vi "zlgcan_demo_CANFDNET_TCP .vi"() -> ()   [LabVIEW 2018]
doc: "适用的设备：CANET-E-U、CANET-2E-U、CANET-4E-U、CANET-8E-U、\nCANET-200T、CANET-100T"
uses:
  data_type/ZCAN_InitCAN_setting_CANET.ctl
  data_type/ZCAN_TransmitFD_Data.ctl
  data_type/ZCAN_Transmit_Data.ctl
panel:
  in  "ZCAN_Transmit_Data":T1
  in  "ZCAN_TransmitFD_Data":T2
  in  "CANFD数据帧数组":T3(array[cluster])
  in  "CAN数据帧数组":T4(array[cluster])
  out "已接收帧数":u32
  out "CAN报文显示":string[][](table)
  out "CANFD报文显示":string[][](table)
  out "error out 2":errorcluster caption="错误输出"
  out "source":string
  in  "ZCAN_InitCAN_setting_CANET":T5
  in  "开启CAN":bool
  in  "stop":bool
  in  "?":T6(tab)
  in  "CAN卡型号":u32(ring)=48 items=["CANFDNET-800U -TCP"=57, "CANFDNET-100U -TCP"=55, "CANFDNET-400U -TCP"=52, "CANFDNET-200U-TCP"=48]
  in  "索引":u32(ring) items=["0", "1", "2", "3", "4", "5", "6", "7", "8"]
  in  "CAN 通道":u32(ring) items=["0", "1", "2", "3"]
  in  "TCP模式":u32(ring) items=["客户端（client）", "服务器（server）"]
  in  "IP":string="192.168.0.178"
  in  "工作端口":u32=4001
  in  "本地端口":u32=8000
  out "设备句柄":u32
  out "通道句柄":u32
  out "error out":errorcluster caption="状态"
  out "数据长度":u8=8 max=8
  in  "CANFD加速？":u32(ring) items=["不加速", "加速"]
  in  "数据输入":string="11 22 33 44 55 66 77 88"
  in  "协议":u32(ring) items=["CAN", "CANFD"]
  in  "发送方式":u32(ring) items=["正常发送", "单次发送", "自发自收", "单次自发自收"]
  in  "帧格式":u32(ring) items=["数据帧", "远程帧"]
  in  "帧类型":u32(ring) items=["标准帧", "扩展帧"]
  in  "ID":u32=18 format="0x%08x"
  in  "发送":bool
  # "适用的设备：CANFDNET-100U -TCP、CANFDNET200U_TCP、CANFDNET-400U -TCP、CANFDNET-800U -TCP"
  # "停止程序前，\n请先关闭CAN卡"
  # "当CANET的工作模式为：\n\n1. 客户端（TCP Client）\n\n   LabVIEW 设备型号选择【 CANFDNET-TCP】\n\n   TCP模式选择【服务器 TCP Sever】\n\n   填写电脑本机IP+本地端口。\n\n2. 服务器（TCP Sever）\n\n   LabVIEW 设备型号选择【 CANFDNET-TCP】\n\n   TCP模式选择【客户端 TCP Client】\n\n   填写CANFDNET的 IP +工作端口\n\n3. UDP\n\n   LabVIEW 设备型号选择【 CANFDNET-UDP】\n\n   填写CANFDNET的IP+工作端口+本地端口"
  # "1. 调试运行DEMO前，将bin文件夹下面的kerneldlls文件夹先拷贝至LabView安装目录，\n如 D:\\Program Files (x86)\\National Instruments\\LabVIEW 2018。"
  # "2. 确保电脑有VC++ 2005/2008/2010/2013运行库（对应32，64位），可到微软官网下载。"
  # "3，如果打开设备失败，可能原因：\n（1）没有进行第二步操作；\n（2）已经打开过一次，没有正常关闭的情况下，继续点击“打开设备”，是无法打开的。\n     需要USB重新拔插，LABVIEW重启（全部关闭），然后再“打开设备”。\n (3) 项目路径不能有中文繁体。"
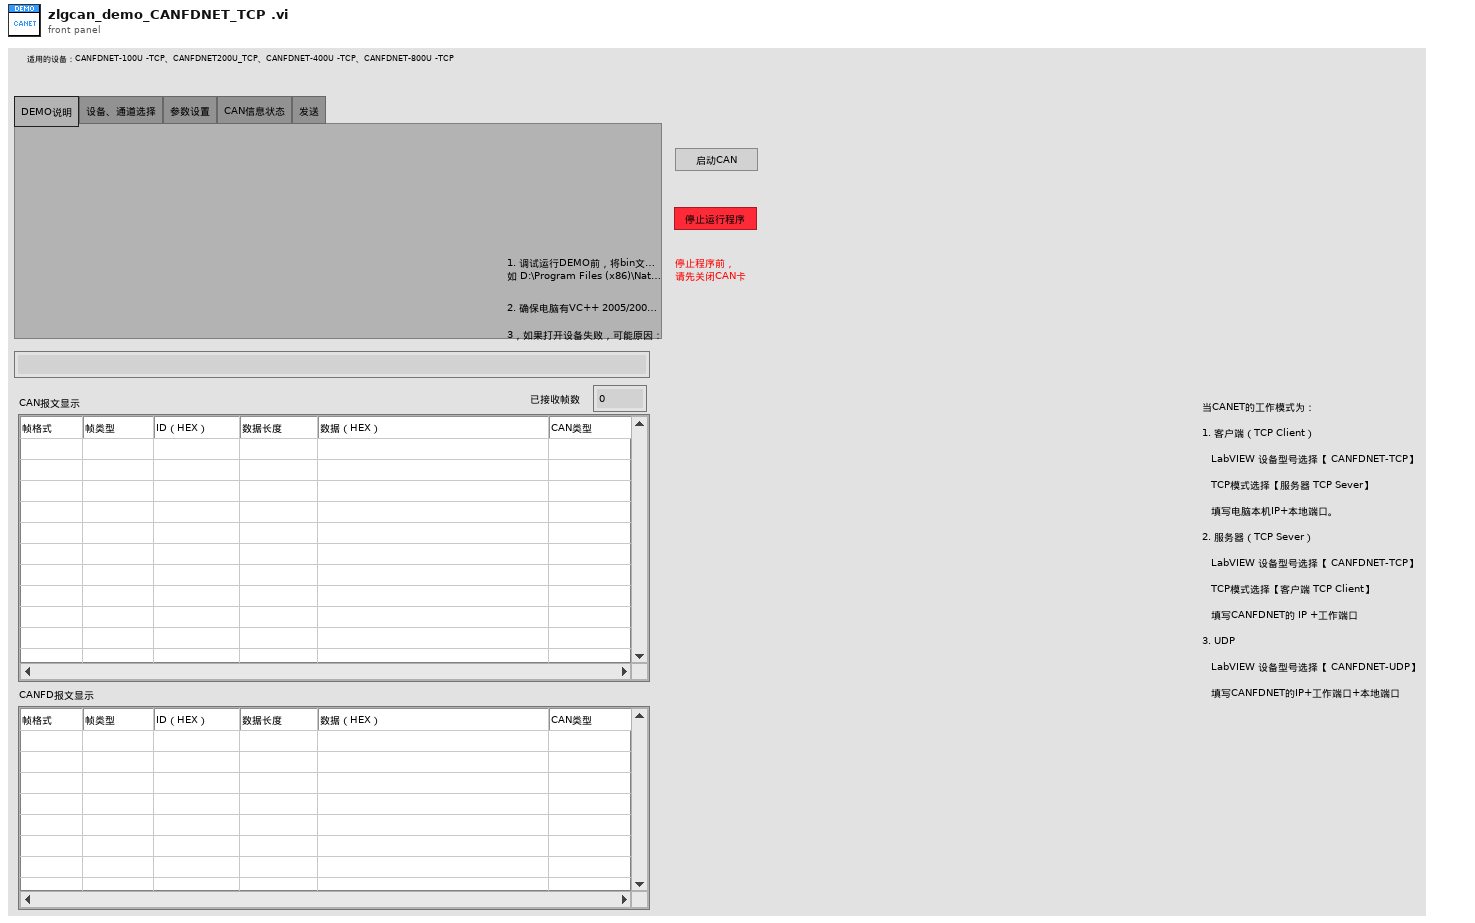
[diagram p1: front panel]
types:
  T1 = typedef "ZCAN_Transmit_Data.ctl" = cluster{"帧类型":u32, "帧格式":u32, "ID":u32, "数据长度":u8, "DATA":cluster{"CAN数据[0]":u8, "CAN数据[1]":u8, "CAN数据[2]":u8, "CAN数据[3]":u8, "CAN数据[4]":u8, "CAN数据[5]":u8, "CAN数据[6]":u8, "CAN数据[7]":u8}, "发送方式":u32}
  T2 = typedef "ZCAN_TransmitFD_Data.ctl" = cluster{"帧类型":u32, "帧格式":u32, "ID":u32, "数据长度":u8, "CANFD加速？":u8, "DATA":cluster{"CAN数据[0]":u8, "CAN数据[1]":u8, "CAN数据[2]":u8, "CAN数据[3]":u8, "CAN数据[4]":u8, "CAN数据[5]":u8, "CAN数据[6]":u8, "CAN数据[7]":u8, "CAN数据[8]":u8, "CAN数据[9]":u8, "CAN数据[10]":u8, "CAN数据[11] ":u8, "CAN数据[12] ":u8, "CAN数据[13] ":u8, "CAN数据[14] ":u8, "CAN数据[15] ":u8, "CAN数据[16]":u8, "CAN数据[17]":u8, "CAN数据[18]":u8, "CAN数据[19]":u8, "CAN数据[20]":u8, "CAN数据[21]":u8, "CAN数据[22]":u8, "CAN数据[23]":u8, "CAN数据[24] ":u8, "CAN数据[25]":u8, "CAN数据[26]":u8, "CAN数据[27]":u8, "CAN数据[28]":u8, "CAN数据[29]":u8, "CAN数据[30]":u8, "CAN数据[31]":u8, "CAN数据[32]":u8, "CAN数据[33]":u8, "CAN数据[34]":u8, "CAN数据[35]":u8, "CAN数据[36]":u8, "CAN数据[37]":u8, "CAN数据[38]":u8, "CAN数据[39]":u8, "CAN数据[40]":u8, "CAN数据[41]":u8, "CAN数据[42]":u8, "CAN数据[43]":u8, "CAN数据[44]":u8, "CAN数据[45]":u8, "CAN数据[46]":u8, "CAN数据[47]":u8, "CAN数据[48]":u8, "CAN数据[49]":u8, "CAN数据[50]":u8, "CAN数据[51]":u8, "CAN数据[52]":u8, "CAN数据[53]":u8, "CAN数据[54]":u8, "CAN数据[55]":u8, "CAN数据[56]":u8, "CAN数据[57]":u8, "CAN数据[58]":u8, "CAN数据[59]":u8, "CAN数据[60]":u8, "CAN数据[61]":u8, "CAN数据[62]":u8, "CAN数据[63]":u8}, "发送方式":u32}
  T3 = cluster{u32, u8, u8, u8, u8, cluster{"[0]":u8, "[1]":u8, "[2]":u8, "[3]":u8, "[4]":u8, "[5]":u8, "[6]":u8, "[7]":u8, "[8]":u8, "[9]":u8, "[10]":u8, "[11]":u8, "[12]":u8, "[13]":u8, "[14]":u8, "[15]":u8, "[16]":u8, "[17]":u8, "[18]":u8, "[19]":u8, "[20]":u8, "[21]":u8, "[22]":u8, "[23]":u8, "[24]":u8, "[25]":u8, "[26]":u8, "[27]":u8, "[28]":u8, "[29]":u8, "[30]":u8, "[31]":u8, "[32]":u8, "[33]":u8, "[34]":u8, "[35]":u8, "[36]":u8, "[37]":u8, "[38]":u8, "[39]":u8, "[40]":u8, "[41]":u8, "[42]":u8, "[43]":u8, "[44]":u8, "[45]":u8, "[46]":u8, "[47]":u8, "[48]":u8, "[49]":u8, "[50]":u8, "[51]":u8, "[52]":u8, "[53]":u8, "[54]":u8, "[55]":u8, "[56]":u8, "[57]":u8, "[58]":u8, "[59]":u8, "[60]":u8, "[61]":u8, "[62]":u8, "[63]":u8}, u64}[]
  T4 = cluster{u32, u8, u8, u8, u8, cluster{"[0]":u8, "[1]":u8, "[2]":u8, "[3]":u8, "[4]":u8, "[5]":u8, "[6]":u8, "[7]":u8}, u64}[]
  T5 = typedef "ZCAN_InitCAN_setting_CANET.ctl" = cluster{"tcp_type":u32, "work_port":u32, "local_port":u32, "IP":string}
  T6 = enum32{"DEMO说明", "设备、通道选择", "参数设置", "CAN信息状态", "发送"}
  T7 = cluster{"[0]":u32, "[1]":u32, "[2]":u32, "[3]":u32, "[4]":u32, "[5]":u32, "[6]":u32, "[7]":u32, "[8]":u32, "[9]":u32, "[10]":u32, "[11]":u32, "[12]":u32, "[13]":u32, "[14]":u32, "[15]":u32, "[16]":u32, "[17]":u32, "[18]":u32, "[19]":u32, "[20]":u32, "[21]":u32, "[22]":u32, "[23]":u32, "[24]":u32, "[25]":u32, "[26]":u32, "[27]":u32, "[28]":u32, "[29]":u32, "[30]":u32, "[31]":u32, "[32]":u32, "[33]":u32, "[34]":u32, "[35]":u32, "[36]":u32, "[37]":u32, "[38]":u32, "[39]":u32, "[40]":u32, "[41]":u32, "[42]":u32, "[43]":u32, "[44]":u32, "[45]":u32, "[46]":u32, "[47]":u32, "[48]":u32, "[49]":u32, "[50]":u32, "[51]":u32, "[52]":u32, "[53]":u32, "[54]":u32, "[55]":u32, "[56]":u32, "[57]":u32, "[58]":u32, "[59]":u32, "[60]":u32, "[61]":u32, "[62]":u32, "[63]":u32}
  T8 = cluster{"[0]":u32, "[1]":u32, "[2]":u32, "[3]":u32, "[4]":u32, "[5]":u32, "[6]":u32, "[7]":u32}
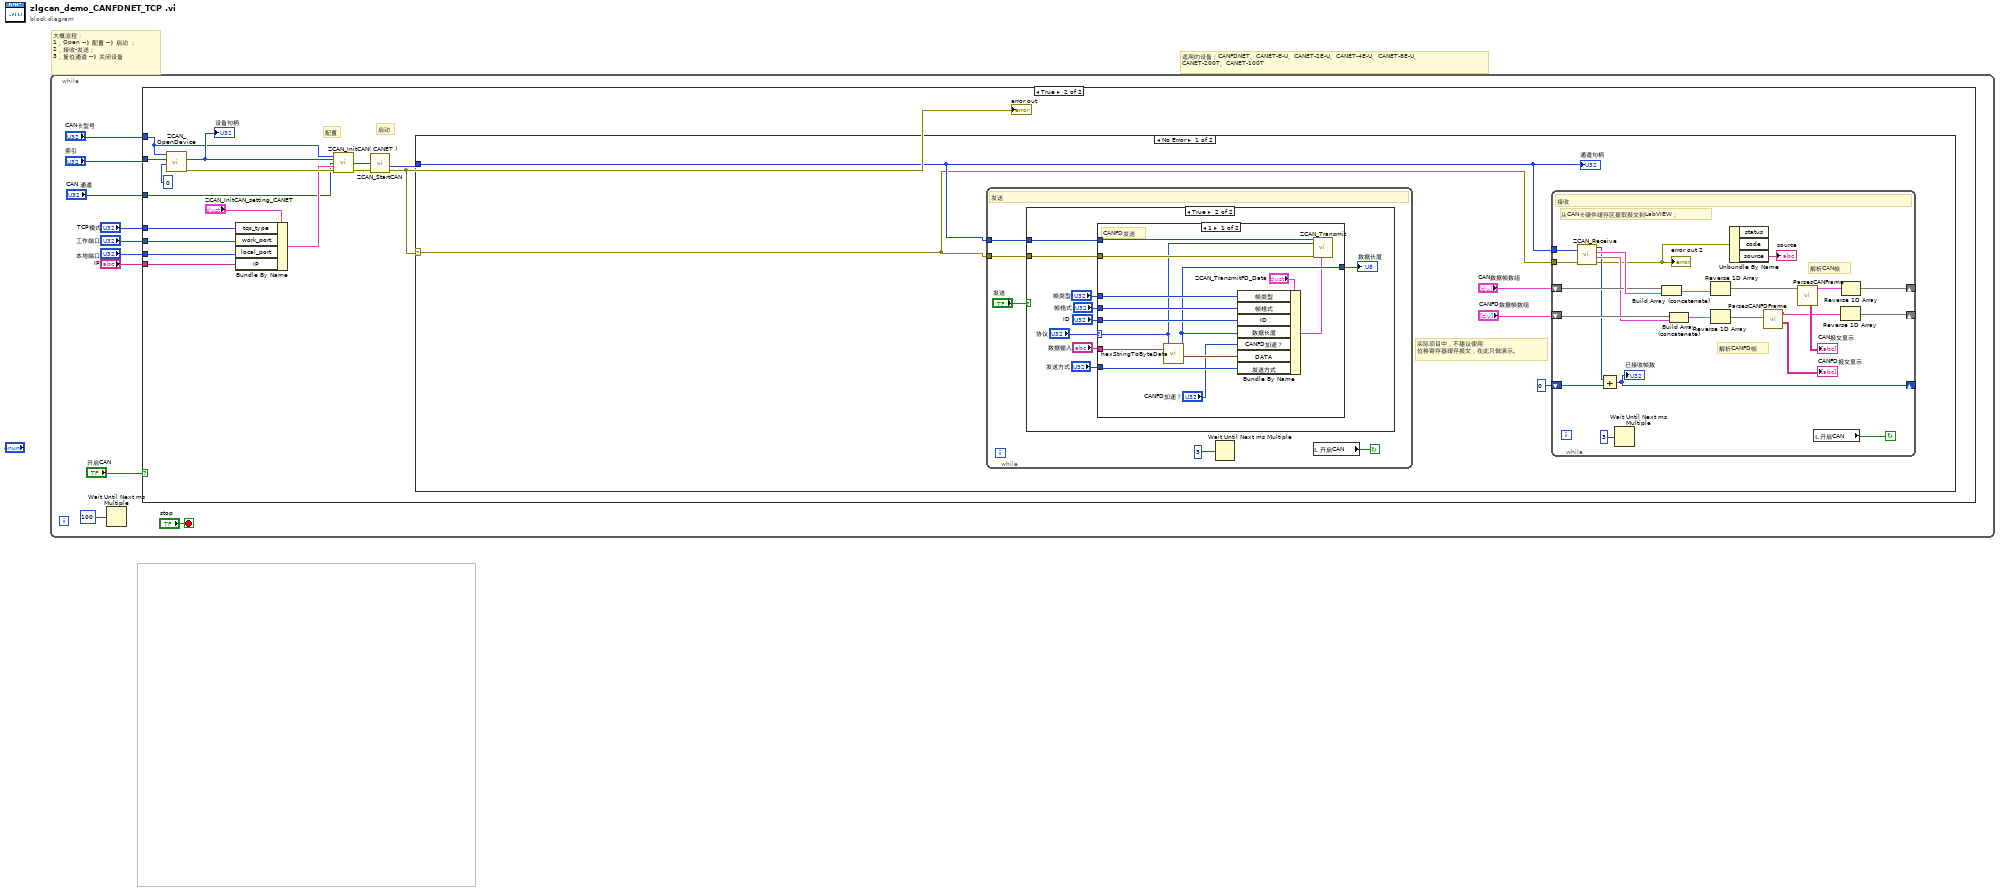
[diagram p0: block diagram]
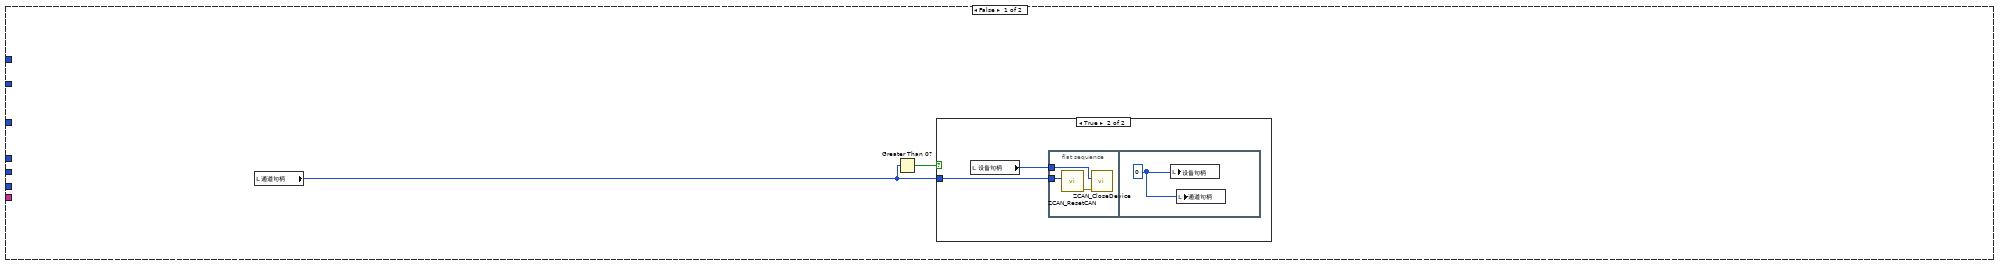
[diagram p2: hidden frame]
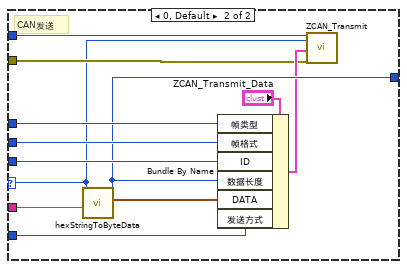
[diagram p5: hidden frame]
diagram:
  # "适用的设备：CANFDNET、CANET-E-U、CANET-2E-U、CANET-4E-U、CANET-8E-U、\nCANET-200T、CANET-100T"
  # "大概流程：\n1，Open --》配置 --》启动 ；\n2，接收-发送；\n3，复位通道 --》关闭设备"
  n1 = while {
    stop <- "stop" stop-if-true
    n2 = Wait Until Next ms Multiple(millisecond multiple=u32 100) -> ()  [unwired: 1 out]
    n3 = case shown="True" "开启CAN" {
      tunnel: "CAN卡型号" -> [_ w21]
      tunnel: "索引" -> [_ w33]
      tunnel: "TCP模式" -> [_ w30]
      tunnel: "工作端口" -> [_ w29]
      tunnel: "本地端口" -> [_ w28]
      tunnel: "IP" -> [_ w27]
      tunnel: "CAN 通道" -> [_ w23]
      frame False {
        # "关闭CAN卡"
        n4 = local read "通道句柄"() -> (w11:u32)
        n5 = Greater Than 0?(x=w11) -> (x > 0?=w12:bool)
        n6 = case shown="True" w12 {
          tunnel: w11 -> [_ w14]
          frame False {
          }
          frame True {
            n7 = local read "设备句柄"() -> (w13:u32)
            n8 = flat-sequence {
              tunnel: w14 -> [w16]
              tunnel: w13 -> [w15]
              frame #0 {
                n9 = call "ZCAN_ResetCAN.vi"("can_handle"=w16) -> ("error out"=w17:errorcluster)  [unwired: 9 in, 1 out]
                n10 = call "ZCAN_CloseDevice.vi"("error in (no error)"=w17, "device_handle"=w15) -> ()  [unwired: 8 in, 2 out]
              }
              frame #1 {
                w18 = u32 0 ("can_index_handle(out)")
                n11 = local write "设备句柄"(w18) -> ()
                n12 = local write "通道句柄"(w18) -> ()
              }
            }
          }
        }
      }
      frame True {
        # "启动"
        # "配置"
        n13 = call "ZCAN_OpenDevice.vi"("reserved"=0, "device_index"=w33, "device_type"=w21) -> ("error out"=w26:errorcluster, "DEVICE_HANDLE"=w22:u32)  [unwired: 7 in]
        "设备句柄" <- w22
        n14 = Bundle By Name(cluster="ZCAN_InitCAN_setting_CANET", "tcp_type"=w30, "work_port"=w29, "local_port"=w28, "IP"=w27) -> (w24:T5)
        n15 = call "ZCAN_InitCAN( CANET ).vi"("设备类型"=w21, "device_hande"=w22, "CANindex"=w23, "ZCAN_InitCAN_setting_CANET"=w24, "error in (no error)"=w26) -> ("can_index_handle"=w20:u32, "error out"=w25:errorcluster)  [unwired: 9 in]
        n16 = call "ZCAN_StartCAN.vi"("error in (no error)"=w25, "can_index_handle"=w20) -> ("error out"=w19:errorcluster, "can_index_handle(out)"=w32:u32)  [unwired: 7 in, 1 out]
        "error out" <- w19
        n17 = case shown="No Error" w19 {
          selector: w19 -> [w35 _]
          tunnel: w32 -> [w36 _]
          frame No Error {
            # "实际项目中，不建议使用\n位移寄存器缓存报文，在此只做演示。"
            n18 = while {
              tunnel: w36 -> [w40]
              tunnel: w35 -> [w41]
              stop <- w42 continue-if-true
              # "发送"
              n19 = case shown="True" "发送" {
                tunnel: w40 -> [_ w46]
                tunnel: w41 -> [_ w47]
                frame False {
                }
                frame True {
                  n20 = case shown="1" "协议" {
                    selector: "协议" -> [w54 w67]
                    tunnel: "帧类型" -> [w65 w77]
                    tunnel: "帧格式" -> [w64 w76]
                    tunnel: "ID" -> [w63 w75]
                    tunnel: "发送方式" -> [w62 w73]
                    tunnel: [w58 w72] -> w48
                    tunnel: "数据输入" -> [w60 w71]
                    tunnel: w47 -> [w57 w69]
                    tunnel: w46 -> [w55 w68]
                    frame 1 {
                      # "CANFD发送"
                      n21 = call "hexStringToByteData.vi"("数据输入"=w60, "协议"=w54) -> ("CANFD_data"=w61:T7, "字节数"=w58:i32)  [unwired: 7 in, 1 out]
                      n22 = Bundle By Name(cluster="ZCAN_TransmitFD_Data", "帧类型"=w65, "帧格式"=w64, "ID"=w63, "数据长度"=w58, "CANFD加速？"="CANFD加速？", "DATA"=w61, "发送方式"=w62) -> (w56:T2)
                      n23 = call "ZCAN_Transmit.vi"("can_index_handle"=w55, "协议"=w54, "error in (no error)"=w57, "ZCAN_TransmitFD_Data"=w56) -> ()  [unwired: 15 in, 1 out]
                    }
                    frame 0, Default {
                      # "CAN发送"
                      n24 = call "hexStringToByteData.vi"("数据输入"=w71, "协议"=w67) -> ("CAN_data"=w74:T8, "字节数"=w72:i32)  [unwired: 7 in, 1 out]
                      n25 = Bundle By Name(cluster="ZCAN_Transmit_Data", "帧类型"=w77, "帧格式"=w76, "ID"=w75, "数据长度"=w72, "DATA"=w74, "发送方式"=w73) -> (w70:T1)
                      n26 = call "ZCAN_Transmit.vi"("can_index_handle"=w68, "协议"=w67, "ZCAN_Transmit_Data"=w70, "error in (no error)"=w69) -> ()  [unwired: 15 in, 1 out]
                    }
                  }
                  "数据长度" <- w48
                }
              }
              n27 = Wait Until Next ms Multiple(millisecond multiple=u32 3) -> ()  [unwired: 1 out]
              n28 = local read "开启CAN"() -> (w42:bool)
            }
            n29 = while {
              tunnel: w35 -> [w99]
              tunnel: w36 -> [w98]
              shift-right: [w100] -> _
              shift-left: 0 -> [w86]
              shift-right: [w90] -> _
              shift-left: "CAN数据帧数组" -> [w96]
              shift-right: [w88] -> _
              shift-left: "CANFD数据帧数组" -> [w94]
              stop <- w79 continue-if-true
              # "从CAN卡硬件缓存区提取报文到LabVIEW；"
              # "解析CANFD帧"
              # "解析CAN帧"
              # "接收"
              n30 = call "ZCAN_Receive.vi"("error in (no error)"=w99, "can_handle"=w98) -> ("error out"=w80:errorcluster, "CANFD数据帧数组"=w93:T3, "CAN数据帧数组"=w97:T4, "Receive_Num"=w87:u32)  [unwired: 2 in]
              "error out 2" <- w80
              n31 = Add(x=w87, y=w86) -> (x+y=w100:u32)
              "已接收帧数" <- w100
              n32 = Wait Until Next ms Multiple(millisecond multiple=u32 3) -> ()  [unwired: 1 out]
              n33 = Build Array (concatenate)(w96, w97) -> (w95:T4)
              n34 = Build Array (concatenate)(w94, w93) -> (w92:T3)
              n35 = Reverse 1D Array(array=w95) -> (reversed array=w89:T4)
              n36 = Reverse 1D Array(array=w92) -> (reversed array=w84:T3)
              n37 = Unbundle By Name(w80) -> ("source"=→"source":string)  [unwired: 2 out]
              n38 = call "ParsesCANFDFrame.vi"("CANFD数据帧数组"=w84) -> ("CANFD报文显示"=→"CANFD报文显示":string[][], "CANFD数据帧数组(out)"=w83:T3)  [unwired: 9 in]
              n39 = call "ParsesCANFrame.vi"("CAN数据帧数组"=w89) -> ("CAN数据帧数组(out)"=w91:T4, "CAN报文显示"=→"CAN报文显示":string[][])  [unwired: 9 in]
              n40 = local read "开启CAN"() -> (w79:bool)
              n41 = Reverse 1D Array(array=w83) -> (reversed array=w88:T3)
              n42 = Reverse 1D Array(array=w91) -> (reversed array=w90:T4)
            }
            "通道句柄" <- w36
          }
          frame Error {
          }
        }
      }
    }
  }
